vi "API - DIO - Disable Digital IO.vi"(8 "error in":errorcluster, 11 "TCP Network Connection in":refnum<k5>) -> (0 "error out":errorcluster, 3 "TCP Network Connection out":refnum<k5>)   [LabVIEW 2020]
doc: "Disabled the digital IO port and sets all digital lines to inputs."
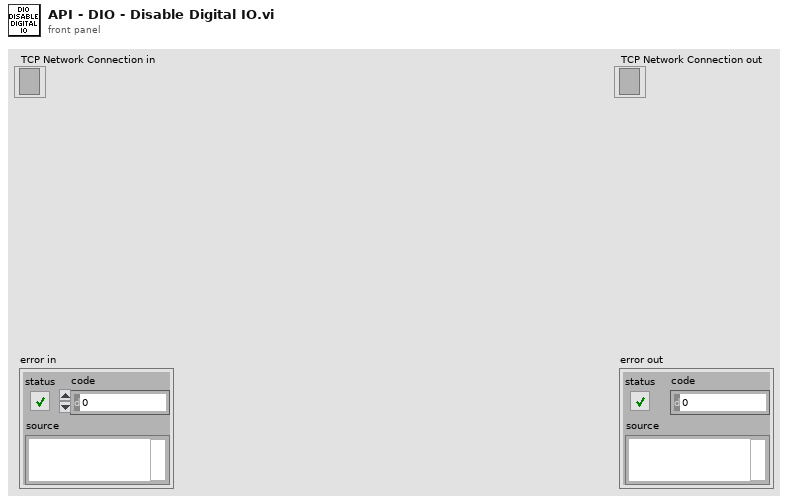
[diagram p1: front panel]
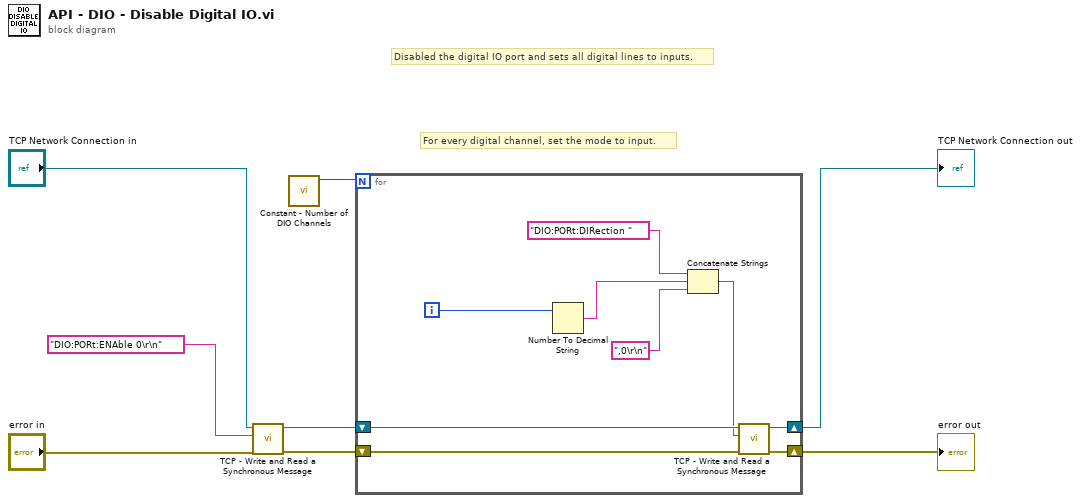
[diagram p0: block diagram]
diagram:
  # "For every digital channel, set the mode to input."
  # "Disabled the digital IO port and sets all digital lines to inputs."
  n1 = call "TCP - Write and Read a Synchronous Message.vi"("error in"="error in", "Message to Send"="DIO:PORt:ENAble 0\r\n", "TCP Network Connection in"="TCP Network Connection in") -> ("error out"=w2:errorcluster, "TCP Network Connection out"=w3:refnum<k5>)  [unwired: 6 in, 1 out]
  n2 = call "Constant - Number of DIO Channels.vi"() -> ("Maximum Channel"=w1:i32)  [unwired: 11 in]
  n3 = for {
    N: w1 -> [_]
    shift-right: [w16] -> w5
    shift-left: w3 -> [w15]
    shift-right: [w17] -> w6
    shift-left: w2 -> [w14]
    i -> [w9]
    n4 = Number To Decimal String(number=w9) -> (decimal integer string=w11:string)  [unwired: 1 in]
    n5 = Concatenate Strings("DIO:PORt:DIRection " ("Message to Send"), w11, ",0\r\n" ("string")) -> (w12:string)
    n6 = call "TCP - Write and Read a Synchronous Message.vi"("error in"=w14, "Message to Send"=w12, "TCP Network Connection in"=w15) -> ("error out"=w17:errorcluster, "TCP Network Connection out"=w16:refnum<k5>)  [unwired: 6 in, 1 out]
  }
  "TCP Network Connection out" <- w5
  "error out" <- w6
